vi "Alp Dev Halt.vi"(8 "error in (no error)":errorcluster, 11 "DeviceId":u32) -> (0 "error out":errorcluster, 3 "function return":i32)   [LabVIEW 2013, in "alpD41.lvlib"]
doc: "ALP_API long ALP_ATTR AlpDevHalt( ALP_ID DeviceId);"
uses:
  <userlib>/alpD41/alpD41.lvlib
  <userlib>/alpD41/alpD41.dll
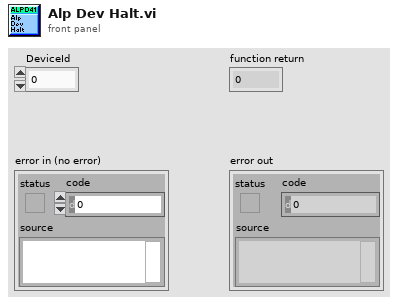
[diagram p1: front panel]
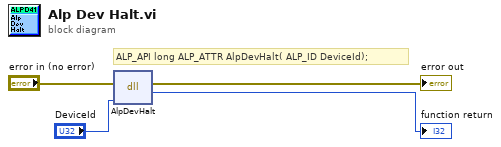
[diagram p0: block diagram]
diagram:
  # "ALP_API long ALP_ATTR AlpDevHalt( ALP_ID DeviceId);"
  n1 = dll-call lib="C:/Program Files (x86)/National Instruments/LabVIEW 2013/user.lib/alpD41/alpD41.*" fn="AlpDevHalt"(error in="error in (no error)", "DeviceId"="DeviceId") -> (error out=→"error out":errorcluster, →"function return":i32)  [unwired: 3 in, 1 out]
